vi "Measure_V_Multi.vi"(8 "errin":errorcluster, 11 "visa in":refnum<visa-resource-name>) -> (0 "errout":errorcluster, 3 "Measurements":dbl[](array[numeric]))   [LabVIEW 2020]
uses:
  <vilib>/Instr/_visa.llb/VISA Open Access Mode.ctl
  C/Program Files (x86)/National Instruments/LabVIEW 2020/instr.lib/Agilent 3446X Series/Public/Data/Read (Single Point).vi
  C/Program Files (x86)/National Instruments/LabVIEW 2020/instr.lib/Agilent 3446X Series/Agilent 3446X Series.lvlib
panel:
  out "Tableau 2":u32[](array[numeric])
  out "Tableau":u32[](array[numeric])
  out "Numérique":i32
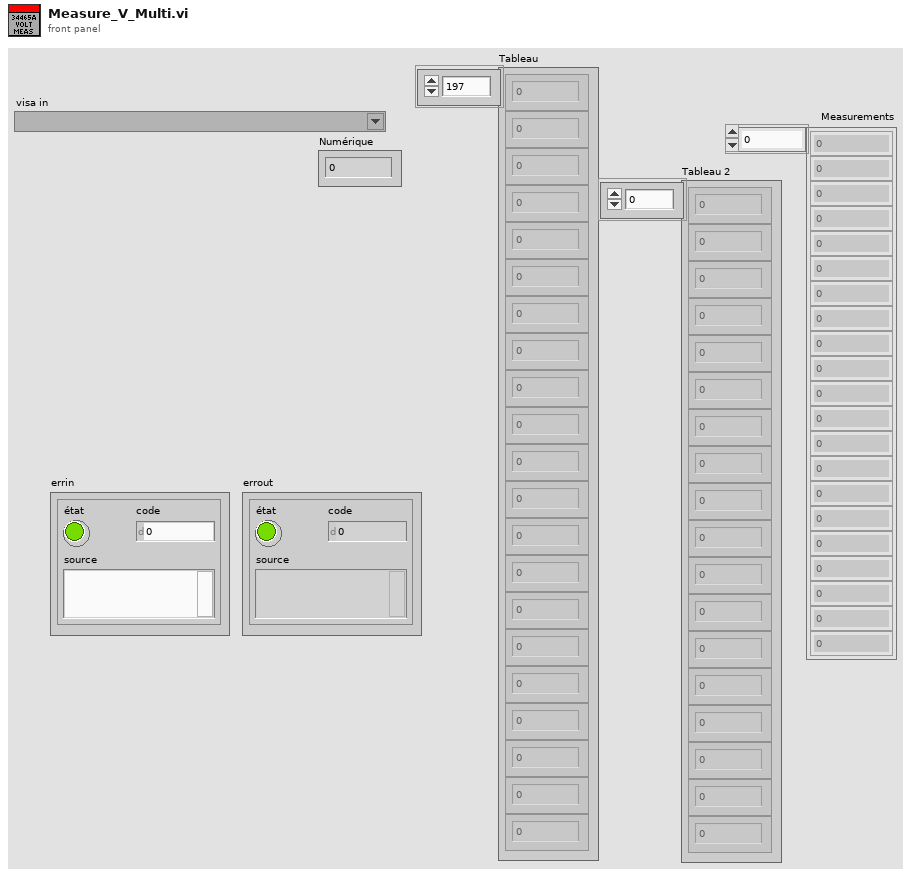
[diagram p1: front panel]
types:
  T1 = typedef "VISA Open Access Mode.ctl" = u32
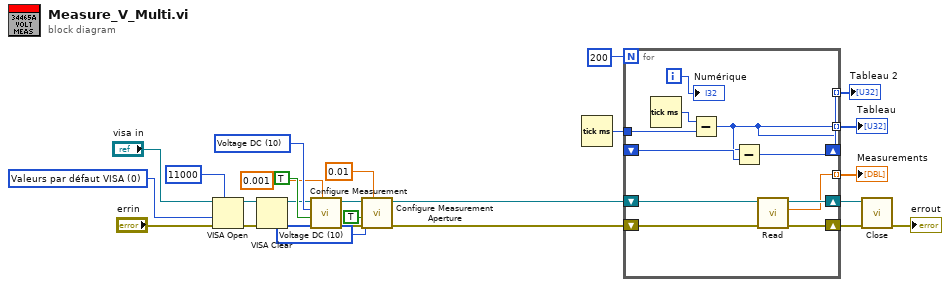
[diagram p0: block diagram]
diagram:
  w5 = 10 items=["Continuity", "Current AC", "Current DC", "Diode", "Frequency", "Resistance 4-wire", "Period", "Resistance 2-wire", "Temperature", "Voltage AC", "Voltage DC", "Voltage DC Ratio", "Capacitance"] ("Measurement Function (0: Continuity)")
  w25 = 10 items=["Continuity", "Current AC", "Current DC", "Diode", "Frequency", "Resistance 4-wire", "Period", "Resistance 2-wire", "Temperature", "Voltage AC", "Voltage DC", "Voltage DC Ratio", "Capacitance"] ("Measurement Function (10: Voltage DC)")
  w19 = T1 0 items=["Valeurs par défaut VISA"=0, "Verrouillage exclusif"=1, "Charger les paramètres configurés"=4] ("Access Mode")
  n1 = VISA Open(timeout (0)=u32 11000 ("Timeout de VISA Open (0)"), access mode=w19, error in (no error)="errin", VISA resource name="visa in") -> (VISA resource name=w17:refnum<visa-resource-name>, error out=w18:errorcluster)  [unwired: 1 out]
  n2 = VISA Clear(VISA resource name=w17, error in (no error)=w18) -> (VISA resource name out=w21:refnum<visa-resource-name>, error out=w22:errorcluster)
  n3 = call "Configure Measurement.vi"("Absolute Resolution (1E-6)"=0.001, "error in (no error)"=w22, "Auto Range (T: Enable)"=TRUE, "Measurement Function (10: Voltage DC)"=w25, "VISA resource name"=w21) -> ("error out"=w7:errorcluster, "VISA resource name out"=w6:refnum<visa-resource-name>)  [unwired: 5 in]
  n4 = call "Configure Measurement Aperture.vi"("Aperture Time (0.1s)"=0.01, "error in (no error)"=w7, "Enable Aperture (F: Disable)"=TRUE, "Measurement Function (0: Continuity)"=w5, "VISA resource name"=w6) -> ("error out"=w1:errorcluster, "VISA resource name out"=w2:refnum<visa-resource-name>)  [unwired: 5 in]
  n5 = Tick Count (ms)() -> (millisecond timer value=w11:u32)
  n6 = for {
    N: 200 ("Timeout (10000 ms)") -> [_]
    shift-right: [w36] -> w23
    shift-left: w1 -> [w35]
    shift-right: [w37] -> w24
    shift-left: w2 -> [w34]
    tunnel: [w27] -> w13 mode=indexing
    tunnel: w11 -> [w31]
    tunnel: [w28] -> w10 mode=indexing
    shift-right: [w28] -> _
    shift-left: _ -> [w30]
    tunnel: [w29] -> w9 mode=indexing
    i -> [w33]
    n7 = Tick Count (ms)() -> (millisecond timer value=w32:u32)
    n8 = Subtract(x=w32, y=w31) -> (x-y=w28:u32)
    n9 = Subtract(x=w28, y=w30) -> (x-y=w29:u32)
    n10 = call-poly "Read.vi"("error in (no error)"=w35, "VISA resource name"=w34) -> ("error out"=w36:errorcluster, "Measurement"=w27:dbl, "VISA resource name out"=w37:refnum<visa-resource-name>)  [unwired: 7 in]
    "Numérique" <- w33
  }
  "Measurements" <- w13
  "Tableau" <- w10
  "Tableau 2" <- w9
  n11 = call "Close.vi"("error in (no error)"=w23, "VISA resource name"=w24) -> ("error out"=→"errout":errorcluster)  [unwired: 9 in]
